vi "Solve Tridiagonal Equations (single right hand DBL).vi"(8 "Known Vector":dbl[](array[numeric]), 9 "Pivot":i32[](array[numeric]), 10 "U":T1, 11 "L":dbl[](array[numeric])) -> (0 "error":i32, 3 "Solution Vector":dbl[](array[numeric]))   [LabVIEW 2017, in "NI_AALPro.lvlib"]
uses:
  NI_AALPro.lvlib
  lvanlys.dll
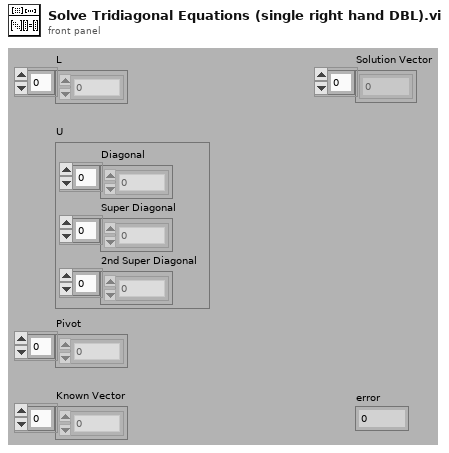
[diagram p1: front panel]
types:
  T1 = cluster{"Diagonal":dbl[], "Super Diagonal":dbl[], "2nd Super Diagonal":dbl[]}
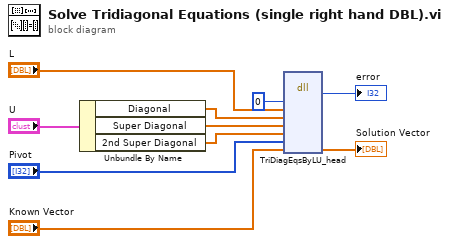
[diagram p0: block diagram]
diagram:
  n1 = Unbundle By Name("U") -> ("Diagonal"=w5:dbl[], "Super Diagonal"=w4:dbl[], "2nd Super Diagonal"=w3:dbl[])
  n2 = dll-call lib="C:/Program Files/National Instruments/LabVIEW 2017/resource/lvanlys.*" fn="TriDiagEqsByLU_head" ("CBLAS.dll:MtrxxVectH")("trans"=0, "SubDiag"="L", "Diag"=w5, "SuperDiag"=w4, "SuperDiag2"=w3, "PVT"="Pivot", "B"="Known Vector") -> ("error"=→"error":i32, "B"=→"Solution Vector":dbl[])  [unwired: 9 in, 2 out]
